vi "startUp.vi"(8 "error in (no error)":errorcluster, 11 "CameraControlViewer in":refnum<class "CameraControlViewer.lvclass">) -> (0 "error out":errorcluster, 3 "CameraControlViewer out":refnum<class "CameraControlViewer.lvclass">)   [LabVIEW 2009, in "Views.lvlib" / "Camera.lvlib" / "CameraControlViewer.lvclass"]
uses:
  CameraControlViewer.lvclass
  CameraControlViewer.lvclass/CameraControlViewer.ctl
  Tools/Filing/FileSystem/FileSystem.lvclass
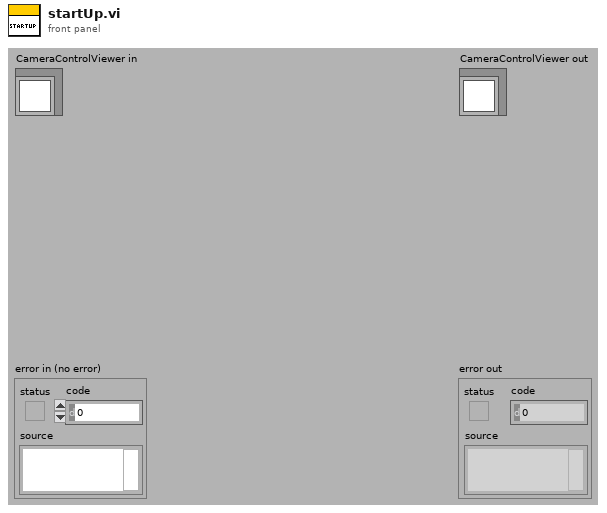
[diagram p1: front panel]
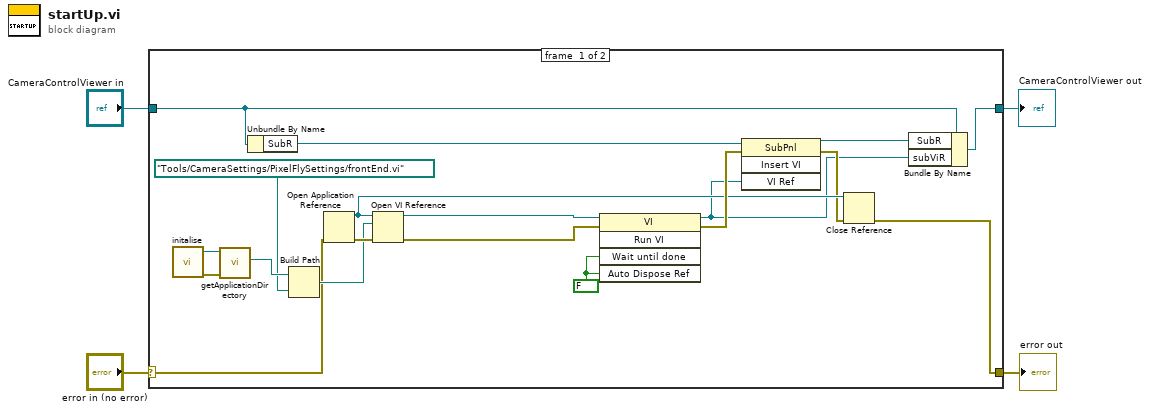
[diagram p0: block diagram]
diagram:
  n1 = case shown="No Error" "error in (no error)" {
    selector: "error in (no error)" -> [w16 w25]
    tunnel: [w8 w25] -> w3
    tunnel: [w10 w24] -> w1
    tunnel: "CameraControlViewer in" -> [w11 w24]
    frame #0 {
      w23 = FALSE
      n2 = call "initalise.vi"() -> ("error out"=w20:errorcluster, "FileSystem out"=w21:refnum<class "FileSystem.lvclass">)  [unwired: 10 in]
      n3 = call-dynamic "getApplicationDirectory.vi"("error in (no error)"=w20, "FileSystem.lvclass in"=w21) -> ("ApplicationDirectory"=w19:path)  [unwired: 7 in, 2 out]
      n4 = Unbundle By Name(w11) -> ("SubR"=w15:refnum<vi>)
      n5 = Build Path(base path=w19, name or relative path=path "Tools/CameraSettings/PixelFlySettings/frontEnd.vi") -> (appended path=w17:path)
      n6 = Open Application Reference(8:w16) -> (0:w22:errorcluster, 3:w13:refnum<vi>)  [unwired: 3 in]
      n7 = Open VI Reference(application reference (local)=w13, vi path=w17, error in (no error)=w22) -> (vi reference=w7:refnum<vi>, error out=w6:errorcluster)  [unwired: 3 in]
      n8 = invoke class="VI" method="Run VI"(reference=w7, error in=w6, "Wait until done"=w23, "Auto Dispose Ref"=w23) -> (reference out=w5:refnum<vi>, error out=w14:errorcluster)  [unwired: 1 in, 3 out]
      n9 = invoke class="SubPnl" method="Insert VI"(reference=w15, error in=w14, "VI Ref"=w5) -> (reference out=w9:refnum<vi>, error out=w12:errorcluster)  [unwired: 1 in, 2 out]
      n10 = Close Reference(reference=w13, error in (no error)=w12) -> (error out=w8:errorcluster)
      n11 = Bundle By Name(cluster=w11, "SubR"=w9, "subViR"=w5) -> (w10:refnum<class "CameraControlViewer.lvclass">)
    }
    frame #1 {
    }
  }
  "error out" <- w3
  "CameraControlViewer out" <- w1
